vi "Get teraterm options.vi"(8 "error in (no error)":errorcluster, 9 "Console number (1)":u32=1 min=1 step=1, 10 "Config name":string, 11 "file (use dialog)":path) -> (0 "error out":errorcluster, 3 "Final teraterm ini string":string)   [LabVIEW 2013]
panel:
  out "Line array":string[](array[string])
  in  "Teraterm ini file template":string="[BG]\n; Use Eterm look-feel Background extension (on/off)\nBGEnable=off\n\n; Use AlphaBlend API (on/off)\nBGUseAlphaBlendAPI=on\n\n; Susie plugin path\nBGSPIPath=plugin\n\n; Fast window sizing/moving\nBGFastSizeMove=on\n\n; Flickerless window moving\nBGFlickerlessMove=on\n\n; If HideTitle=on and BGNoFrame=on, use window without frame\n; you can resize window with Alt + Shift + LeftDrag\nBGNoFrame=on\n\n; wildcard => random select\nBGThemeFile=theme\\*.ini\n\n\n[Tera Term]\n;\tTera Term version number\nVersion=2.3\n\n;\tLanguage (English/Japanese/Russian/Korean/UTF-8)\nLanguage=UTF-8\n\n; User interface language file that includes message strings.\n; Tera Term uses built-in English message when the file or message is not found.\nUILanguageFile=lang\\Default.lng\n\n; Connecting timeout value(per seconds). No action if the value is zero.\n; Connecting socket could be canceled after the value timeout if the value is greater than zero.\n; The default value is zero(depends on Windows TCP/IP stack implementation).\nConnectingTimeout=0\n\n; pasting string by clicking mouse right button disabled\nDisablePasteMouseRButton=off\n\n; pasting string by clicking mouse middle button disabled\nDisablePasteMouseMButton=on\n\n; confirm pasting string by clicking mouse right button\nConfirmPasteMouseRButton=off\n\n; confirm changing clipboard string by clicking mouse right button\nConfirmChangePaste=on\nConfirmChangePasteCR=on\nPasteDialogSize=330,220\nConfirmChangePasteStringFile=\n\n; Scroll out the current buffer when the clear screen does.\nScrollWindowClearScreen=on\n\n; Reset scrollback on display activity\nAutoScrollOnlyInBottomLine=on\n\n; Starting the selection only by a left button.\nSelectOnlyByLButton=on\n\n; Duplicate session by Alt-D Accelerator key disabled\nDisableAcceleratorDuplicateSession=off\n\n; Send break by Alt-B Accelerator key disabled\nDisableAcceleratorSendBreak=off\n\n; Duplicate session Menu disabled\nDisableMenuDuplicateSession=off\n\n; New connection Menu disabled\nDisableMenuNewConnection=off\n\n; Send break Menu disabled\nDisableMenuSendBreak=off\n\n;\tANSI color definition (in the case FullColor=on)\n;\t* UseTextColor should be off, or the background and foreground color of\n;\t  VTColor are assigned to color-number 0 and 7 respectively, even if\n;\t  they are specified in ANSIColor.\n;\t* ANSIColor is a set of 4 values that are color-number(0--15),\n;\t  red-value(0--255), green-value(0--255) and blue-value(0--255).\nANSIColor=0,0,0,0, 1,255,0,0, 2,0,255,0, 3,255,255,0, 4,128,128,255, 5,255,0,255, 6,0,255,255, 7,255,255,255, 8,64,64,64, 9,192,0,0, 10,0,192,0, 11,192,192,0, 12,64,64,192, 13,192,0,192, 14,0,192,192, 15,192,192,192\n; xterm\n; ANSIColor=0,0,0,0, 1,255,0,0, 2,0,255,0, 3,255,255,0, 4,92,92,255, 5,255,0,255, 6,0,255,255, 7,255,255,255, 8,127,127,127, 9,205,0,0, 10,0,205,0, 11,205,205,0, 12,0,0,238, 13,205,0,205, 14,0,205,205, 15,229,229,229\n; PuTTY\n;ANSIColor=0,0,0,0, 1,255,85,85, 2,85,255,85, 3,255,255,85, 4,85,85,255, 5,255,85,255, 6,85,255,255, 7,255,255,255, 8,85,85,85, 9,187,0,0, 10,0,187,0, 11,187,187,0, 12,0,0,187, 13,187,0,187, 14,0,187,187, 15,187,187,187\n; Tera Term Pro 2.3\n;ANSIColor=0,0,0,0, 1,255,0,0, 2,0,255,0, 3,255,255,0, 4,0,0,255, 5,255,0,255, 6,0,255,255, 7,255,255,255, 8,128,128,128, 9,128,0,0, 10,0,128,0, 11,128,128,0, 12,0,0,128, 13,128,0,128, 14,0,128,128, 15,192,192,192\n; Solarized (http://ethanschoonover.com/solarized)\n;ANSIColor=0,7,54,66, 1,203,75,22, 2,88,110,117, 3,101,123,131, 4,131,148,150, 5,108,113,196, 6,147,161,161, 7,253,246,227, 8,0,43,54, 9,220,50,47, 10,133,153,0, 11,181,137,0, 12,38,139,210, 13,211,54,130, 14,42,161,152, 15,238,232,213\n\n;\tEnable continued-line copy\nEnableContinuedLineCopy=on\n\n; Mouse cursor type (arrow/ibeam/cross/hand)\nMouseCursor=ibeam\n\n; Translucent window (0 - 255: transparency value)\nAlphaBlend=255\n\n; Cygwin install path\nCygwinDirectory=c:\\cygwin\n\n; Viewlog Editor path\nViewlogEditor=C:\\Windows\\notepad.exe\n\n; Locale for Unicode\n;Locale=chs\nLocale=american\n\n; CodePage for Unicode\nCodePage=65001\n\n; Background color of text uses background color of screen (on/off)\nUseNormalBGColor=on\n\n;\tPort type (serial/tcpip/namedpipe)\nPort=???\n\n;\tWindow positions\nVTPos=-2147483648,-2147483648\nTEKPos=-2147483648,-2147483648\n\n;\tTerminal size\nTerminalSize=115,45\n;\tTerminal size=window size (on/off)\nTermIsWin=on\n;\tAuto window resizing option (on/off)\nAutoWinResize=off\n\n;\tConvert a received new-line (CR) char to CR/CRLF/LF/AUTO\nCRReceive=AUTO\n;\tNew-line code to be transmitted (CR/CRLF)\nCRSend=CR\n\n;\tTerminal ID\nTerminalID=VT100\n\n;\tLocal echo (on/off)\nLocalEcho=off\n\n;\tAnswerback\nAnswerback=\n\n;\tAuto window switching (VT<->TEK; on/off)\nAutoWinSwitch=off\n\n;\tKanji code to be received (SJIS/EUC/JIS)\nKanjiReceive=UTF-8\n;\tJIS Katakana code to be received (7/8)\nKatakanaReceive=8\n\n;\tKanji code to be transmitted (SJIS/EUC/JIS)\nKanjiSend=UTF-8\n;\tJIS Katakana to be transmitted (7/8)\nKatakanaSend=8\n;\tKanji-in sequence to be transmitted (@/B)\nKanjiIn=B\n;\tKanji-out sequence to be transmitted (J/B)\nKanjiOut=J\n\n;\tRussian code set used in host\nRussHost=Windows\n;\tRussian code set used in PC\nRussClient=Windows\n\n;\tWindow title\nTitle=Teraterm\n\n;\tCursor shape (block/vertical/horizontal)\nCursorShape=block\n\n;\tHide title & menu bars and enable popup menu (on/off)\nHideTitle=off\n;\tHide menu bar and enable popup menu (on/off)\nPopupMenu=off\n\n;\tColor mode (on/off)\nEnableANSIColor=on\nPcBoldColor=on\nAixterm16Color=on\nXterm256Color=on\n\n;\tEnable scroll buffer (on/off)\nEnableScrollBuff=on\n;\tScroll buffer size\nScrollBuffSize=10000\n\n;  \tText and background colors\n;\t\tfor Normal characters\nVTColor=255,255,255,0,0,0\n;\tSolarized Dark\n;VTColor=131,148,150,0,43,54\n;\tSolarized Light\n;VTColor=101,123,131,253,246,227\n;\n;\t\tfor Bold characters\nEnableBoldAttrColor=on\nVTBoldColor=255,255,0,0,0,0\n;\tSolarized Dark\n;VTBoldColor=147,161,161,7,54,66\n;\tSolarized Light\n;VTBoldColor=88,110,117,238,232,213\n;\n;\t\tfor Blink characters\nEnableBlinkAttrColor=on\nVTBlinkColor=255,0,0,0,0,0\n;\tSolarized Dark\n;VTBlinkColor=133,153,0,0,43,54\n;\tSolarized Light\n;VTBlinkColor=133,153,0,253,246,227\n;\n;\t\tfor Reverse characters\nEnableReverseAttrColor=on\nVTReverseColor=0,0,0,255,255,255\n;\tSolarized Dark\n;VTReverseColor=0,43,54,131,148,150\n;VTReverseColor=101,123,131,253,246,227\n;\tSolarized Light\n;VTReverseColor=253,246,227,101,123,131\n;VTReverseColor=131,148,150,0,43,54\n;\n;\t\tfor URL(hyper link) text color\nEnableURLColor=on\nURLUnderline=on\nURLColor=0,255,255,0,0,0\n;\tSolarized Dark\n;URLColor=181,137,0,0,43,54\n;\tSolarized Light\n;URLColor=181,137,0,253,246,227\n;\n\n; Enable clickable URL\nEnableClickableUrl=on\n\n; Launched Browser\n;   Firefox example\n;     ClickableUrlBrowser=firefox\n;     ClickableUrlBrowserArg=-new-tab\n;   Opera example\n;     ClickableUrlBrowser=opera\n;     ClickableUrlBrowserArg=-newpage\n;   IE example\n;     ClickableUrlBrowser=iexplore\n;     ClickableUrlBrowserArg=\n;   Chrome example\n;     ClickableUrlBrowser=chrome\n;     ClickableUrlBrowserArg=\nClickableUrlBrowser=\nClickableUrlBrowserArg=\n\n\n;\t\tfor TEK window\nTEKColor=0,0,0,255,255,255\n\n;\tTEK color emulation (on/off)\nTEKColorEmulation=off\n\n;\tFont\nVTFont=Terminal,0,-19,0\n;\tBold style font (on/off)\nEnableBold=off\n;\tFont for TEK window\nTEKFont=Terminal,0,-8,255\n;\tFont quality(default/non-antialiased/antialiased/cleartype)\nFontQuality=default\n\n;\tRussian code set of the font\nRussFont=Windows\n\n;\tBackspace key (BS/DEL)\nBSKey=BS\n;\ttransmit DEL by Delete key (on/off)\nDeleteKey=on\n\n;\tRussian code set used in the keyboard driver\nRussKeyb=Windows\n\n;\tMeta key (on/off/left/right)\nMetaKey=off\n\n;\tMeta key sets MSB (off/raw/text)\nMeta8Bit=off\n\n;\tApplication keypad mode disabled.\nDisableAppKeypad=off\n\n;\tApplication cursor mode disabled.\nDisableAppCursor=off\n\n;\tSerial port parameters\n;\t  Port number\nComPort=TheComPort\n;\t  Baud rate\nBaudRate=115200\n;\t  Parity (even/odd/none/mark/space)\nParity=none\n;\t  Data (7/8)\nDataBit=8\n;\t  Stop (1/1.5/2)\nStopBit=1\n;\t  Flow control (x/hard/none)\nFlowCtrl=none\n;\t  Transmit delay per character (in msec)\nDelayPerChar=0\n;\t  Transmit delay per line (in msec)\nDelayPerLine=0\n\n;\tTCP/IP parameters\n;\t  TCP port#\nTCPPort=22\n;\t  Telnet flag (on/off)\nTelnet=on\n;\t  Telnet terminal type\n;TermType=vt100\nTermType=xterm\n\n;\t  Auto window closing option (on/off)\nAutoWinClose=on\n;\t  History list of hosts\nHistoryList=on\n\n; Binary flag for Send File (on/off)\nTransBin=off\n\n; without transfer dialog flag for Send File (on/off)\nFTHideDialog=off\n\n; Binary flag for Log (on/off)\nLogBinary=off\n; Log append (on/off)\nLogAppend=on\n; plain text flag for Log (on/off)\nLogTypePlainText=on\n; timestamp flag for Log (on/off)\nLogTimestamp=off\n; without transfer dialog flag for Log (on/off)\nLogHideDialog=off\n; Current all buffer included in first (on/off)\nLogIncludeScreenBuffer=off\n\n; Default Log file name. You can specify strftime format to here.\nLogDefaultName=teraterm.log\n; Default path to save the log file.\nLogDefaultPath=\n; Auto start logging with default log file name.\nLogAutoStart=off\n\n; === Log Rotate ===\n; Mode: 0(none), 1(size)\nLogRotate=0\n; Size\nLogRotateSize=0\n; Size type: 0(byte), 1(KB), 2(MB)\nLogRotateSizeType=0\n; Step: 0(none), >=1(count times)\nLogRotateStep=0\n\n; Deferred Log Write Mode (on/off)\nDeferredLogWriteMode=on\n\n\n; XMODEM option (checksum/crc/1k)\nXmodemOpt=checksum\n; Binary flag for XMODEM Receive and ZMODEM Send (on/off)\nXmodemBin=on\n\n; XMODEM receive command\nXmodemRcvCommand=\n\n; Default directory for file transfers\nFileDir=C:\\Program Files (x86)\\teraterm\n\n; Filter for send file\nFileSendFilter=\n\n; SCP sending directory\nScpSendDir=~/\n\n; Save Broadcast Command History\nBroadcastCommandHistory=on\n\n; Broadcast command enabling flag on the dialog window (on/off)\nAcceptBroadcast=on\n\n; Number of broadcast command history\nMaxBroadcatHistory=99\n\n;------ special options (see Tera Term help)\n\n; C1 (8-bit) control characters\nAccept8BitCtrl=on\nSend8BitCtrl=off\n\n; Accept remote-controlled window title changing (off/overwrite/ahead/last)\nAcceptTitleChangeRequest=overwrite\n\n; Wrong kanji-out ^[(H (Japanese only)\nAllowWrongSequence=off\n\n; Alternate screen buffer support\nAlternateScreenBuffer=on\n\n; Auto file renaming for downloading\nAutoFileRename=on\n\n; Auto text copying\nAutoTextCopy=on\n\n; Back wrap\nBackWrap=off\n\n; Beep by BEL (on/off/visual)\nBeep=on\n\n; Beep over-used\nBeepOverUsedTime=2\nBeepOverUsedCount=5\nBeepSuppressTime=5\n\n; Beep on connection & disconnection\nBeepOnConnect=off\n\n; B-Plus auto receive\nBPAuto=off\n\n; Escape all control characters in B-Plus\nBPEscCtl=off\n\n; B-Plus log\nBPLog=off\n\n; Clear serial port buffer when port opening\nClearComBuffOnOpen=on\n\n; Clear screen when window is resized\nClearOnResize=on\n\n; Clear screen after the connection is closed\nClearScreenOnCloseConnection=off\n\n; Clipboard access from remote (on/off/read/write)\nClipboardAccessFromRemote=off\n\n; \"Disconnect?\" warning\nConfirmDisconnect=on\n\n; Control characters in kanji (Japanese only)\nCtrlInKanji=on\n\n; Confirm send a file when drag and drop\nConfirmFileDragAndDrop=on\n\n; allow the sequences related to cursor control\nCursorCtrlSequence=off\n\n; Display all characters (debug mode)\nDebug=off\n; Debug mode type which can be selected by user.\n;   on|all   = All types\n;   off|none = Disabled debug mode\n;   normal   = usual teraterm debug mode\n;   hex      = hex output\n;   noout    = disable output completely\nDebugModes=all\n\n; Delimters for word selection\n;  (compatible with earlier versions of Tera Term)\n;  DelimList=$20\n;  DelimDBCS=off\nDelimList=$20!\"#$24%&'()*+,:;<=>?@[\\]^`{|}\nDelimDBCS=on\n\n; Disable mouse event tracking when Control-Key is pressed.\nDisableMouseTrackingByCtrl=on\n\n; Disable wheel to cursor translation when Control-Key is pressed.\nDisableWheelToCursorByCtrl=on\n\n; Line at a time mode\nEnableLineMode=on\n\n; Popup menu\nEnablePopupMenu=on\n\n; \"Show menu bar\" command\nEnableShowMenu=on\n\n; Enable the status line\nEnableStatusLine=on\n\n; Display \"New Connection\" dialog on startup\nHostDialogOnStartup=on\n\n; Enable IME / inline input (Japanese only)\nIME=on\nIMEInline=on\n\nIMERelatedCursor=off\n\n; Windows 7 jump list support\nJumpList=on\n\n; Join Split URL\nJoinSplitURL=off\nJoinSplitURLIgnoreEOLChar=\\\n\n; Kermit log\nKmtLog=off\n; Kermit CAPAS: Ability to transmit and receive extended-length packets\nKmtLongPacket=off\n; Kermit CAPAS: Ability to accept \"A\" packets (file attributes)\nKmtFileAttr=off\n\n; Language selection\nLanguageSelection=on\n\n; Lock Terminal Unique ID\nLockTUID=on\n\n; Exclusive lock for log file\nLogLockExclusive=on\n\n; Max scroll buffer size\nMaxBuffSize=500000\n\n; Max serial port number\nMaxComPort=256\n\n; Max buffer size of OSC string\nMaxOSCBufferSize=4096\n\n; Mouse event tracking\nMouseEventTracking=on\n\n; Maximized window bug tweak\nMaximizedBugTweak=on\n\n; Nonblinking cursor\nNonblinkingCursor=off\n\n; Polygon cursor for KILLFOCUS\nKillFocusCursor=on\n\n; Delay for pass-thru printing (in secs)\nPassThruDelay=3\n\n; Direct pass-thru printing\nPassThruPort=\n\n; Delay for paste per each lines (in msec)\nPasteDelayPerLine=10\n\n; Allow the sequences related to printer control\nPrinterCtrlSequence=on\n\n; Printer font\nPrnFont=\n\n; Page margins for printing\n; (left, right, top and bottom in 1/100 inches)\nPrnMargin=50,50,50,50\n\n; Quick-VAN log\nQVLog=off\n\n; Quick-VAN window size\nQVWinSize=8\n\n; Russian code set of printer font\nRussPrint=Windows\n\n; Save VT Window position\nSaveVTWinPos=off\n\n; Max lines per one jump scroll\nScrollThreshold=12\n\n; Scroll line count with mouse wheel button\nMouseWheelScrollLine=3\n\n; Text selection on window activation\nSelectOnActivate=on\n\n; Startup macro\nStartupMacro=\n\n; Strict Key Mapping\nStrictKeyMapping=off\n\n; Tab Stop Modify Sequence (on/off/combination of HTS,HTS7,HTS8,TBC,TBC0,TBC3)\nTabStopModifySequence=on\n\n; TEK mouse code\nTEKGINMouseCode=32\n\n; Telnet Auto Detection\nTelAutoDetect=on\n\n; Telnet binary option\nTelBin=off\n\n; Telnet auto echo\nTelEcho=off\n\n; Telnet log\nTelLog=off\n\n; Standard telnet port\nTelPort=23\n\n; Keep-Alive packet sending interval on telnet connection (per second, 0=disabled)\nTelKeepAliveInterval=300\n\n; Auto setup for non-telnet\nTCPLocalEcho=off\nTCPCRSend=\n\n; Terminal Unique ID\nTerminalUID=FFFFFFFF\n\n; Title format\n; format ID:  5(000101) <title> - <host/port> VT/TEK\n; format ID: 13(001101) <host/port> - <title> VT/TEK\n; format ID: 29(011101) <host:tcpport/port> - <title> VT/TEK\n; format ID: 45(101101) <host/port:baud> - <title> VT/TEK\n; format ID: 61(111101) <host:tcpport/port:baud> - <title> VT/TEK\nTitleFormat=61\n\n; Allow the sequences related to title report (accept/ignore/empty)\nTitleReportSequence=empty\n\n; Translate mouse wheel to cursor key when application cursor mode\nTranslateWheelToCursor=on\n\n; Unknown Unicode character handling\nUnknownUnicodeCharacterAsWide=off\n\n; Mapping of Unicode to DEC special character\n;   The sum of following values:\n;   1 : Box drawings (U+2500-U+257F)\n;   2 : Bullet (U+2022)\n;       Hyphenation point (U+2027)\n;       Light shade (25%) (U+2591)\n;       Medium shade (50%) (U+2592)\n;       Dark shade (75%) (U+2593)\n;       Black small square (U+25AA)\n;       Black vertical rectangle (U+25AE)\n;       Black verty small square (U+2B1D)\n;   4 : Middle dot (U+00B7)\n;       One dot leader (U+2024)\n;       Bullet operator (U+2219)\nUnicodeToDecSpMapping=3\n\n; White & black color conversion\nUseTextColor=off\n\n; VT Compatible Tab\nVTCompatTab=off\n\n; Space between characters (lines)\nVTFontSpace=0,0,0,0\n\n; Window Icon\nVTIcon=Default\nTEKIcon=Default\n\n; Scaling factors for printing (in pixels per inch)\nVTPPI=0,0\nTEKPPI=0,0\n\n; `wait4all' macro command\nWait4allMacroCommand=off\n\n; allow the sequences related to window control\nWindowCtrlSequence=on\n\n; allow the sequences related to window report\nWindowReportSequence=on\n\n; [Window] menu\nWindowMenu=on\n\n; XMODEM log\nXmodemLog=off\n\n; YMODEM log\nYmodemLog=off\n\n; YMODEM receive command\nYmodemRcvCommand=\n\n; ZMODEM auto receive\nZmodemAuto=off\n\n; ZMODEM parameters for sending\nZmodemDataLen=1024\nZmodemWinSize=32767\n\n; Escape all control characters in ZMODEM\nZmodemEscCtl=off\n\n; ZMODEM log\nZmodemLog=off\n\n; ZMODEM receive command\nZmodemRcvCommand=rz\n\n;------ end of special options\n\n[TTSSH]\n; SSH enabled flag (1=enabled 0=disabled)\nEnabled=1\n\n; default login username (setup to authentication dialog)\nDefaultUserName=\nDefaultForwarding=\n\n; Cipher algorithm order\n;  2...DES(SSH1),    3...3DES(SSH1),   6...Blowfish(SSH1), 7...3DES-CBC,\n;  8...AES128-CBC,   9...AES192-CBC,   :...AES256-CBC,     ;...Blowfish-CBC,\n;  <...AES128-CTR,   =...AES192-CTR,   >...AES256-CTR,     ?...Arcfour,\n;  @...Arcfour128,   A...Arcfour256,   B...CAST128-CBC,    C...3DES-CTR,\n;  D...Blowfish-CTR, E...CAST128-CTR,  F...Camellia128-CBC,\n;  G...Camellia192-CBC, H...Camellia256-CBC, I...Camellia128-CTR,\n;  J...Camellia192-CTR, K...Camellia256-CTR\n;  0...Ciphers below this line are disabled.\nCipherOrder=K>H:J=G9I<F8C7D;A@?EB3062\n\n; KEX algorithm order(SSH2)\n;  0...diffie-hellman-group1-sha1\n;  1...diffie-hellman-group14-sha1\n;  2...diffie-hellman-group-exchange-sha1\n;  3...diffie-hellman-group-exchange-sha256\n;  4...ecdh-sha2-nistp256\n;  5...ecdh-sha2-nistp384\n;  6...ecdh-sha2-nistp521\n;  7...KEXs below this line are disabled.\nKexOrder=56743210\n\n; Host Key algorithm order(SSH2)\n;  2...RSA\n;  3...DSA\n;  4...ecdh-sha2-nistp256\n;  5...ecdh-sha2-nistp384\n;  6...ecdh-sha2-nistp521\n;  7...ED25519\n;  0...below this line are disabled.\nHostKeyOrder=4567230\n\n; MAC algorithm order(SSH2)\n;  1...hmac-sha1\n;  2...hmac-md5\n;  3...hmac-sha1-96\n;  4...hmac-md5-96\n;  5...hmac-ripemd160@openssh.com\n;  6...hmac-sha2-256\n;  8...hmac-sha2-512\n;  0...below this line are disabled.\nMacOrder=86152034\n\n; Compression algorithm order(SSH2)\n;  1...none\n;  2...zlib\n;  3...zlib@openssh.com(Delayed Compression)\n;  0...below this line are disabled.\nCompOrder=3210\n; packet compression level (0=none)\nCompression=0\n\n\nKnownHostsFiles=ssh_known_hosts\nDefaultRhostsLocalUserName=\nDefaultRhostsHostPrivateKeyFile=\nDefaultRSAPrivateKeyFile=\nDefaultAuthMethod=3\n; Debug message logging level of `TTSSH.LOG'.\n; The default value is disabled(0).\n;   LOG_LEVEL_FATAL      5\n;   LOG_LEVEL_ERROR      10\n;   LOG_LEVEL_URGENT     20\n;   LOG_LEVEL_WARNING    30\n;   LOG_LEVEL_VERBOSE    100\n;   LOG_LEVEL_SSHDUMP    200\nLogLevel=0\nWriteBufferSize=2097152\n\n; SSH protocol version (1 or 2)\nProtocolVersion=2\n\n; SSH heartbeat(keepalive): per second (0=disabled)\nHeartBeat=60\n\n; Remember password in memory (1=enabled 0=disabled)\nRememberPassword=1\n\n; Check supported auth methods with \"none\" method (1=enabled 0=disabled)\nCheckAuthListFirst=0\n\n; Enable connection to the server that has RSA key length less than 768 bit (1=enabled 0=disabled)\nEnableRsaShortKeyServer=0\n\n; SSH agent forwarding (pageant) (1=enabled 0=disabled)\nForwardAgent=0\n\n; Confirm SSH agent forwarding (1=enabled 0=disabled)\nForwardAgentConfirm=1\n\n; Verify host key by DNS (1=enabled 0=disabled)\nVerifyHostKeyDNS=0\n\n; SSH Icon\nSSHIcon=Default\n\n[TTProxy]\nConnectionTimeout=\"10\"\nSocksResolve=\"auto\"\nTelnetHostnamePrompt=\">> Host name: \"\nTelnetUsernamePrompt=\"Username:\"\nTelnetPasswordPrompt=\"Password:\"\nTelnetConnectedMessage=\"-- Connected to \"\nTelnetErrorMessage=\"!!!!!!!!\"\n\n[TTXKanjiMenu]\nUseOneSetting=on\n\n[TTXttyrec]\nRecordStartSize=on\n\n[TTXRecurringCommand]\nEnable=off\nCommand=\nInterval=300\n\n[Resize Menu]\n; 80x62\n;ResizeMenu1= 80, 24\n;\n; 120x52\n;ResizeMenu2=120, 52\n;\n; Width: no-change, Height: 52\n;ResizeMenu3=  0, 52\n;\n; Width: 80, Height: no-change\n;ResizeMenu4= 80,  0\n\n;------ Telnet host list\n;\tMax number of hosts is 200.\n;\tYou can edit this list in the [Setup] TCP/IP dialog box.\n;[Hosts]\n;\tHost name\n;Host1=myhost.example.com\n;\tIPv4 address\n;Host2=192.0.2.1\n;\tIPv6 address\n;Host3=[2001:db8:1:2:8401:02ff:fe03:0405]\n;\tIPv6 address with interface number\n;Host4=[fe80::8401:02ff:fe03:0405%3]\n;\tHost name with option\n;Host5=myhost.example.com /F=myhost.ini\n;\tHost name with user, port and option\n;Host6=user@myhost.example.com:10022 /ssh\n;\tURL\n;Host7=ssh://user@myhost.example.com\n;\tCOM1 port\n;Host8=/C=1\n;\tReplay a file\n;Host9=/R=readme.txt\n\n[Hosts]\nHost1=myhost.example.com\nHost2=192.0.2.1\nHost3=[2001:db8:1:2:8401:2ff:fe03:405]\nHost4=[fe80::8401:2ff:fe03:405%3]\nHost5=myhost.example.com /F=myhost.ini\nHost6=user@myhost.example.com:10022 /ssh\nHost7=ssh://user@myhost.example.com\nHost8=/C=1 ;serial port\nHost9=\\\\.\\pipe\\vmware-serial-port ;Named pipe\nHost10=/R=readme.txt ;replay a file\n"
  out "Info block":string
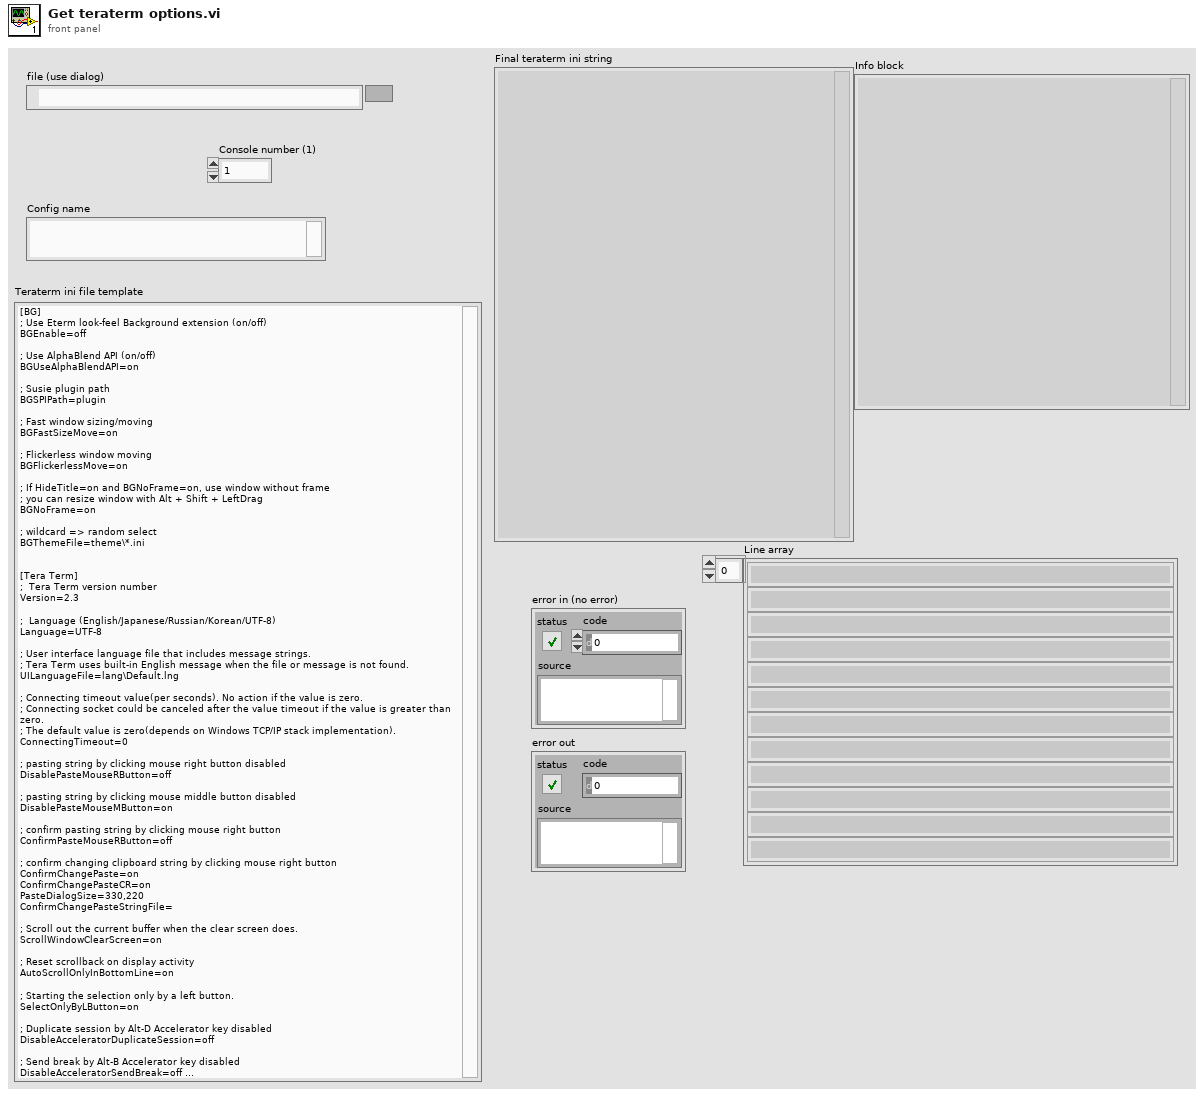
[diagram p1: front panel]
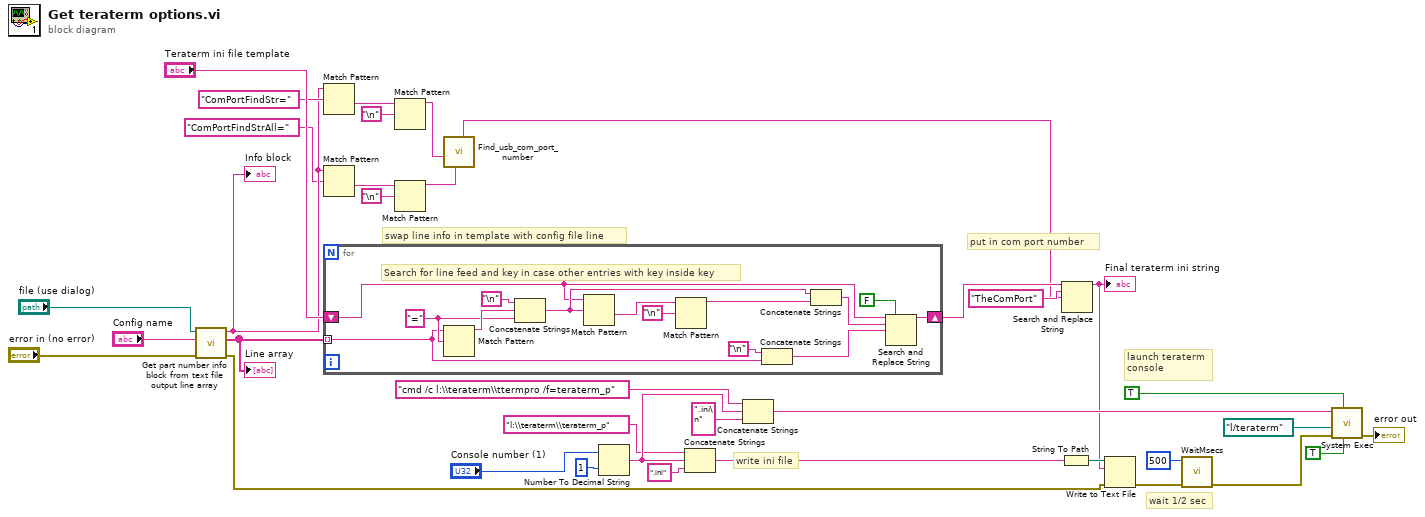
[diagram p0: block diagram]
diagram:
  # "write ini file"
  # "put in com port number"
  # "launch teraterm\nconsole"
  # "wait 1/2 sec"
  # "swap line info in template with config file line"
  n1 = call "Get part number info block from text file output line array.vi"("error in (no error)"="error in (no error)", "Key word"="Config name", "file (use dialog)"="file (use dialog)") -> ("error out"=w1:errorcluster, "Line array"=w33:string[], "Info block"=w25:string)  [unwired: 6 in]
  "Info block" <- w25
  "Line array" <- w33
  n2 = Match Pattern(string=w25, regular expression="ComPortFindStr=") -> (after substring=w30:string)  [unwired: 1 in, 3 out]
  n3 = Match Pattern(string=w25, regular expression="ComPortFindStrAll=") -> (after substring=w26:string)  [unwired: 1 in, 3 out]
  n4 = for {
    tunnel: w33 -> [w42] mode=indexing
    shift-right: [w44] -> w22
    shift-left: "Teraterm ini file template" -> [w39]
    w49 = "=" ("regular expression")
    # "Search for line feed and key in case other entries with key inside key"
    n5 = Match Pattern(string=w42, regular expression=w49) -> (before substring=w50:string)  [unwired: 1 in, 3 out]
    n6 = Concatenate Strings("\n", w50, w49) -> (w46:string)
    n7 = Match Pattern(string=w39, regular expression=w46) -> (after substring=w48:string)  [unwired: 1 in, 3 out]
    n8 = Match Pattern(string=w48, regular expression="\n") -> (before substring=w45:string)  [unwired: 1 in, 3 out]
    n9 = Concatenate Strings("\n", w42) -> (w40:string)
    n10 = Concatenate Strings(w46, w45) -> (w38:string)
    n11 = Search and Replace String(replace all?=FALSE ("replace all? (F)"), input string=w39, search string=w38, replace string=w40) -> (result string=w44:string)  [unwired: 4 in, 3 out]
  }
  n12 = Match Pattern(string=w30, regular expression="\n") -> (before substring=w28:string)  [unwired: 1 in, 3 out]
  n13 = Match Pattern(string=w26, regular expression="\n") -> (before substring=w23:string)  [unwired: 1 in, 3 out]
  n14 = call "Find_usb_com_port_number.vi"("Search key for all output"=w23, "Use this string instead"=w28) -> ("Com port number"=w20:string)  [unwired: 4 in, 5 out]
  n15 = Number To Decimal String(number="Console number (1)", width (-)=i16 1) -> (decimal integer string=w16:string)
  n16 = Concatenate Strings("l:\\teraterm\\teraterm_p", w16, ".ini") -> (w18:string)
  n17 = Concatenate Strings("cmd /c l:\\teraterm\\ttermpro /f=teraterm_p", w16, ".ini\n") -> (w13:string)
  n18 = String To Path(string=w18) -> (path=w19:path)
  n19 = Search and Replace String(input string=w22, search string="TheComPort", replace string=w20) -> (result string=w3:string)  [unwired: 5 in, 3 out]
  "Final teraterm ini string" <- w3
  n20 = Write to Text File(file (use dialog)=w19, text=w3, error in=w1) -> (error out=w7:errorcluster)  [unwired: 1 in, 2 out]
  n21 = call "WaitMsecs.vi"("error in (no error)"=w7, "Wait Msecs"=u32 500) -> ("error out"=w9:errorcluster)  [unwired: 9 in]
  n22 = call <vilib>:"System Exec.vi"("run minimized? (F)"=TRUE, "wait until completion? (T)"=TRUE, "error in (no error)"=w9, "working directory"=path "l:/teraterm", "command line"=w13) -> ("error out"=→"error out":errorcluster)  [unwired: 3 in, 3 out]
